vi "Init_LotObj.vi"(8 "error in (no error)":errorcluster, 11 "WaferTable_Ref":refnum<vi>) -> (0 "error out":errorcluster, 2 "Shutdown":bool, 3 "LotData out":refnum<class "LotData.lvclass">)   [LabVIEW 2012, in "LotData.lvclass"]
uses:
  LotData.lvclass
  Controls/WaferTable.ctl
  Controls/TestData.ctl
  Controls/Measurement.ctl
  Controls/MeasurementType.ctl
  Controls/LotData_Current.ctl
  LotData.lvclass/LotData.ctl
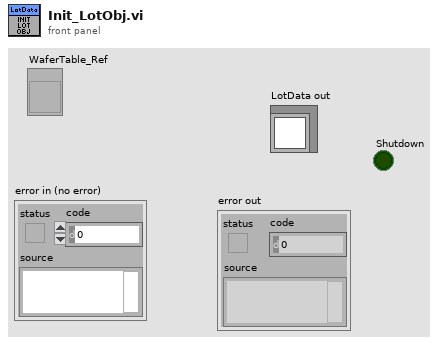
[diagram p1: front panel]
types:
  T1 = typedef "MeasurementType.ctl" = enum16{"Initial", "Final"}
  T2 = cluster{"Area":string, "Wavelength":dbl[], "EL Spectrum":dbl[]}
  T3 = typedef "TestData.ctl" = cluster{"20mA Data":T4, "50mA Data ":T4}
  T4 = typedef "Measurement.ctl" = cluster{"Area":string, "Pad":string, "Current,mA":dbl, "Power":dbl, "WL":dbl, "Voltage":dbl, "Knee Current":dbl, "Reverse":dbl}
  T5 = typedef "LotData.lvclass/LotData_Current.ctl" = cluster{"area":i32, "Data":cluster{"wl":dbl, "power":dbl, "voltage":dbl, "knee":dbl, "reverse":dbl}}
  T6 = typedef "WaferTable.ctl" = string[][]
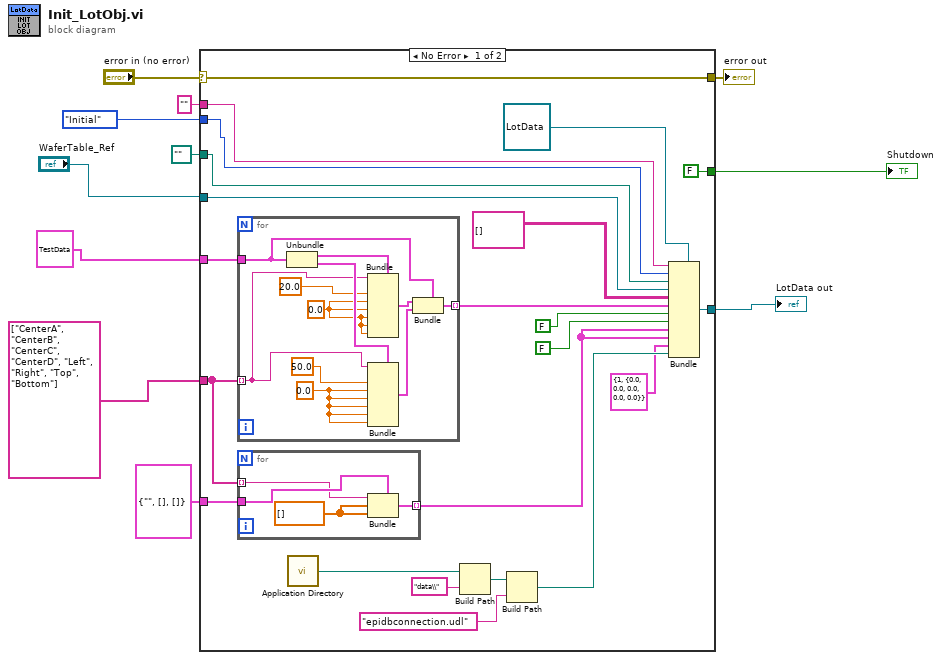
[diagram p0: block diagram]
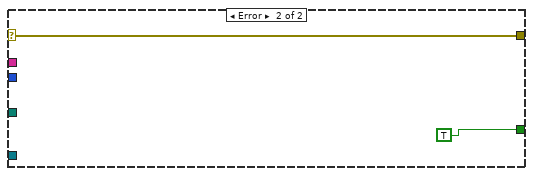
[diagram p2: hidden frame]
diagram:
  n1 = case shown="No Error" "error in (no error)" {
    selector: "error in (no error)" -> [w16 w50]
    tunnel: [w16 w50] -> w10
    tunnel: [w31 _] -> w9
    tunnel: "" ("Wafer ID") -> [w33 _]
    tunnel: path "" ("FilePath") -> [w32 _]
    tunnel: string[] ["CenterA", "CenterB", "CenterC", "CenterD", "Left", "Right", "Top", "Bottom"] -> [w24 _]
    tunnel: "WaferTable_Ref" -> [w29 _]
    tunnel: T3 {"20mA Data"={"Area"="", "Pad"="", "Current,mA"=0.0, "Power"=0.0, "WL"=0.0, "Voltage"=0.0, "Knee Current"=0.0, "Reverse"=0.0}, "50mA Data "={"Area"="", "Pad"="", "Current,mA"=0.0, "Power"=0.0, "WL"=0.0, "Voltage"=0.0, "Knee Current"=0.0, "Reverse"=0.0}} ("TestData") -> [w25 _]
    tunnel: T2 {"Area"="", "Wavelength"=[], "EL Spectrum"=[]} ("Spect") -> [w23 _]
    tunnel: [FALSE ("Shutdown") TRUE ("Shutdown")] -> w3
    tunnel: MeasurementType."Initial" ("Measurement Type") -> [w12 _]
    frame No Error {
      n2 = for {
        tunnel: w25 -> [w45]
        tunnel: w24 -> [w46] mode=indexing
        tunnel: [w42] -> w30 mode=indexing
        w39 = 0.0 ("Power")
        w40 = 0.0 ("Power")
        n3 = Unbundle(w45) -> ("20mA Data"=w48:T4, "50mA Data"=w47:T4)
        n4 = Bundle(cluster=w48, "Area"=w46, "Current,mA"=20.0, "Power"=w40, "WL"=w40, "Voltage"=w40, "Knee Current"=w40, "Reverse"=w40) -> (w44:T4)  [unwired: 1 in]
        n5 = Bundle(cluster=w47, "Area"=w46, "Current,mA"=50.0, "Power"=w39, "WL"=w39, "Voltage"=w39, "Knee Current"=w39, "Reverse"=w39) -> (w43:T4)  [unwired: 1 in]
        n6 = Bundle(cluster=w45, "20mA Data"=w44, "50mA Data"=w43) -> (w42:T3)
      }
      n7 = for {
        tunnel: w24 -> [w36] mode=indexing
        tunnel: w23 -> [w37]
        tunnel: [w34] -> w22 mode=indexing
        w35 = dbl[] [] ("Wavelength")
        n8 = Bundle(cluster=w37, "Area"=w36, "Wavelength"=w35, "EL Spectrum"=w35) -> (w34:T2)
      }
      n9 = call <vilib>:"Application Directory.vi"() -> ("Application Directory"=w21:path)
      n10 = Build Path(base path=w21, name or relative path="data\\") -> (appended path=w19:path)
      n11 = Build Path(base path=w19, name or relative path="epidbconnection.udl") -> (appended path=w17:path)
      n12 = Bundle(cluster=refnum<class "LotData.lvclass"> refnum ("LotData out"), w33, w12, w32, w29, T6 [] ("WaferTable"), w30, FALSE ("Loaded"), FALSE ("Saved"), w22, w22, T5 {"area"=1, "Data"={"wl"=0.0, "power"=0.0, "voltage"=0.0, "knee"=0.0, "reverse"=0.0}} ("Current"), w17) -> (w31:refnum<class "LotData.lvclass">)
    }
    frame Error {
    }
  }
  "error out" <- w10
  "LotData out" <- w9
  "Shutdown" <- w3
